vi "PIDController_Execute.vi"(4 "PID Error Tolerance":T2={"PositionTolerance"=0.001, "VelocityTolerance"=9.9e+30}, 6 "Period":dbl=0.02, 7 "PID Input Limits":T1, 8 "Reset":bool, 9 "SP-SetPoint":dbl, 10 "PV-Measurement":dbl, 11 "PID Tuning":T3={"Kp"=0.0, "Ki"=0.0, "Kd"=0.0, "MaximumIntegral"=9.9e+30, "MinimumIntegral"=-9.9e+30}) -> (0 "AtSetpoint":bool, 1 "CO-ControlOutput":dbl, 3 "out PID_CONTROLLER":T4={"Kp"=0.0, "Ki"=0.0, "Kd"=0.0, "Period"=0.0, "Max_Integral"=0.0, "Min_Integral"=0.0, "Max_Input"=0.0, "Min_Input"=0.0, "Continuous"=FALSE, "PositionError"=0.0, "VelocityError"=0.0, "PrevError"=0.0, "TotalError"=0.0, "PositionTolerance"=0.0, "VelocityTolerance"=0.0, "SetPoint"=0.0, "Kf"=0.0, "Prev_Deriv"=0.0, "Prev_Deriv 2"=0.0, "DerivativeFilter"=FALSE, "Min_Output"=-9.99e+35, "Max_Output"=9.9e+35, "Prev_F_P"=0.0, "Prev_F_P_2"=0.0, "AntiWindupActive"=FALSE} {"Prev_F_P_2" format="%16_6e"; "Prev_F_P" format="%16_6e"; "Max_Output" format="%16_6e"; "Min_Output" format="%16_6e"; "Prev_Deriv 2" format="%16_6e"; "Prev_Deriv" format="%16_6e"; "Kf" format="%16_6e"; "SetPoint" format="%16_6e"; "VelocityTolerance" format="%16_6e"; "PositionTolerance" format="%16_6e"; "TotalError" format="%16_6e"; "PrevError" format="%16_6e"; "VelocityError" format="%16_6e"; "PositionError" format="%16_6e"; "Min_Input" format="%16_6e"; "Max_Input" format="%16_6e"; "Min_Integral" format="%16_6e"; "Max_Integral" format="%16_6e"; "Period" format="%16_6e"; "Kd" format="%16_6e"; "Ki" format="%16_6e"; "Kp" format="%16_6e"})   [LabVIEW 2019, in "Trajectory_Library.lvlib"]
doc: "Convience, single call, LabVIEW function. Creates and calculates the PID controller. Call this routine periodically to calculate the newest output for the provided inputs. \n \nInputs:\n - PID Input Limits -- Cluster containing:\n - MaxInput -- (Default: 0)\n - MinInput -- (Default: 0)\n - Continous -- When True indicates that the input is continuous. (Default: False)\n - PID Tuning -- PID Tuning parameters containing:\n - Kp -- The proportional coefficient.\n - Ki -- The integral coefficient.\n - Kd -- The derivative coefficient.\n - Maximum Integral -- The maximum value of the integrator.\n - Minimum Integral -- The minimum value of the integrator.\n - PV-measurement The current measurement of the process variable. (PV)\n - SP-setpoint The new setpoint of the controller. (SP)\n - Reset -- When True, causes the PID to be reset. (Default: False)\n - Period -- Period of repeated calls in seconds. (Default: 0.020)\n - PID Error Tolerance -- Tolerances for determining \"At Setpoint\", contains:\n - Position Tolerance -- (Default: 0.001)\n - Velocity Tolerance -- (Default: 9.9E+30)\nOutputs:\n - PID_Controller -- Updated PID_Controller data cluster\n - CO-ControlOutput -- Controller output (CO) \n - AtSetpoint -- True when PV is within the specified tolerances of the SP."
uses:
  Trajectory_Library.lvlib
  PID_CONTROLLER.ctl
  PID_TUNING.ctl
  PID_INPUT_LIMITS.ctl
  PID_ERROR_TOLERANCE.ctl
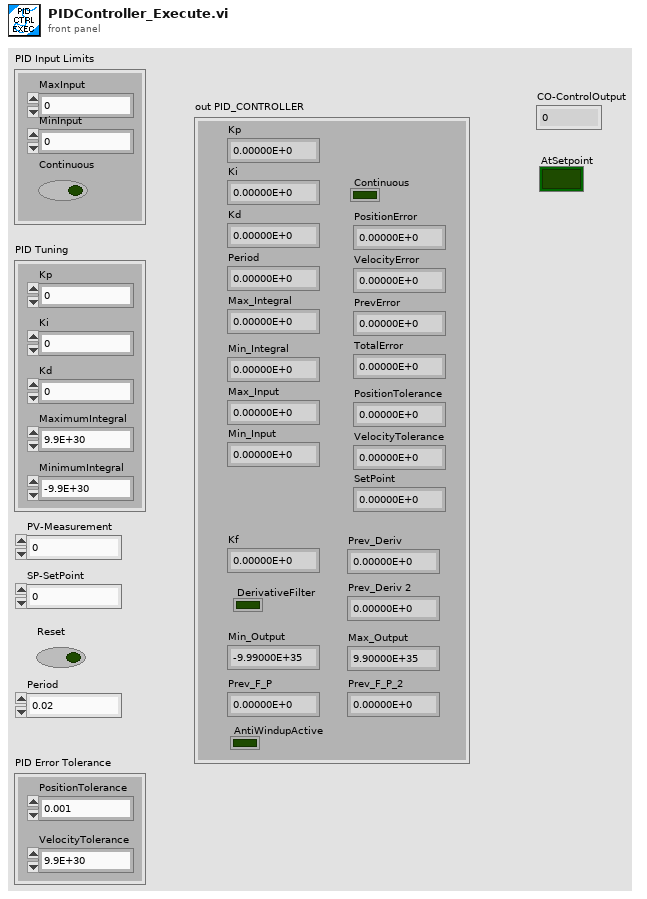
[diagram p1: front panel]
types:
  T1 = typedef "Trajectory_Library.lvlib/PID_INPUT_LIMITS.ctl" = cluster{"MaxInput":dbl, "MinInput":dbl, "Continuous":bool}
  T2 = typedef "Trajectory_Library.lvlib/PID_ERROR_TOLERANCE.ctl" = cluster{"PositionTolerance":dbl, "VelocityTolerance":dbl}
  T3 = typedef "Trajectory_Library.lvlib/PID_TUNING.ctl" = cluster{"Kp":dbl, "Ki":dbl, "Kd":dbl, "MaximumIntegral":dbl, "MinimumIntegral":dbl}
  T4 = typedef "Trajectory_Library.lvlib/PID_CONTROLLER.ctl" = cluster{"Kp":dbl, "Ki":dbl, "Kd":dbl, "Period":dbl, "Max_Integral":dbl, "Min_Integral":dbl, "Max_Input":dbl, "Min_Input":dbl, "Continuous":bool, "PositionError":dbl, "VelocityError":dbl, "PrevError":dbl, "TotalError":dbl, "PositionTolerance":dbl, "VelocityTolerance":dbl, "SetPoint":dbl, "Kf":dbl, "Prev_Deriv":dbl, "Prev_Deriv 2":dbl, "DerivativeFilter":bool, "Min_Output":dbl, "Max_Output":dbl, "Prev_F_P":dbl, "Prev_F_P_2":dbl, "AntiWindupActive":bool}
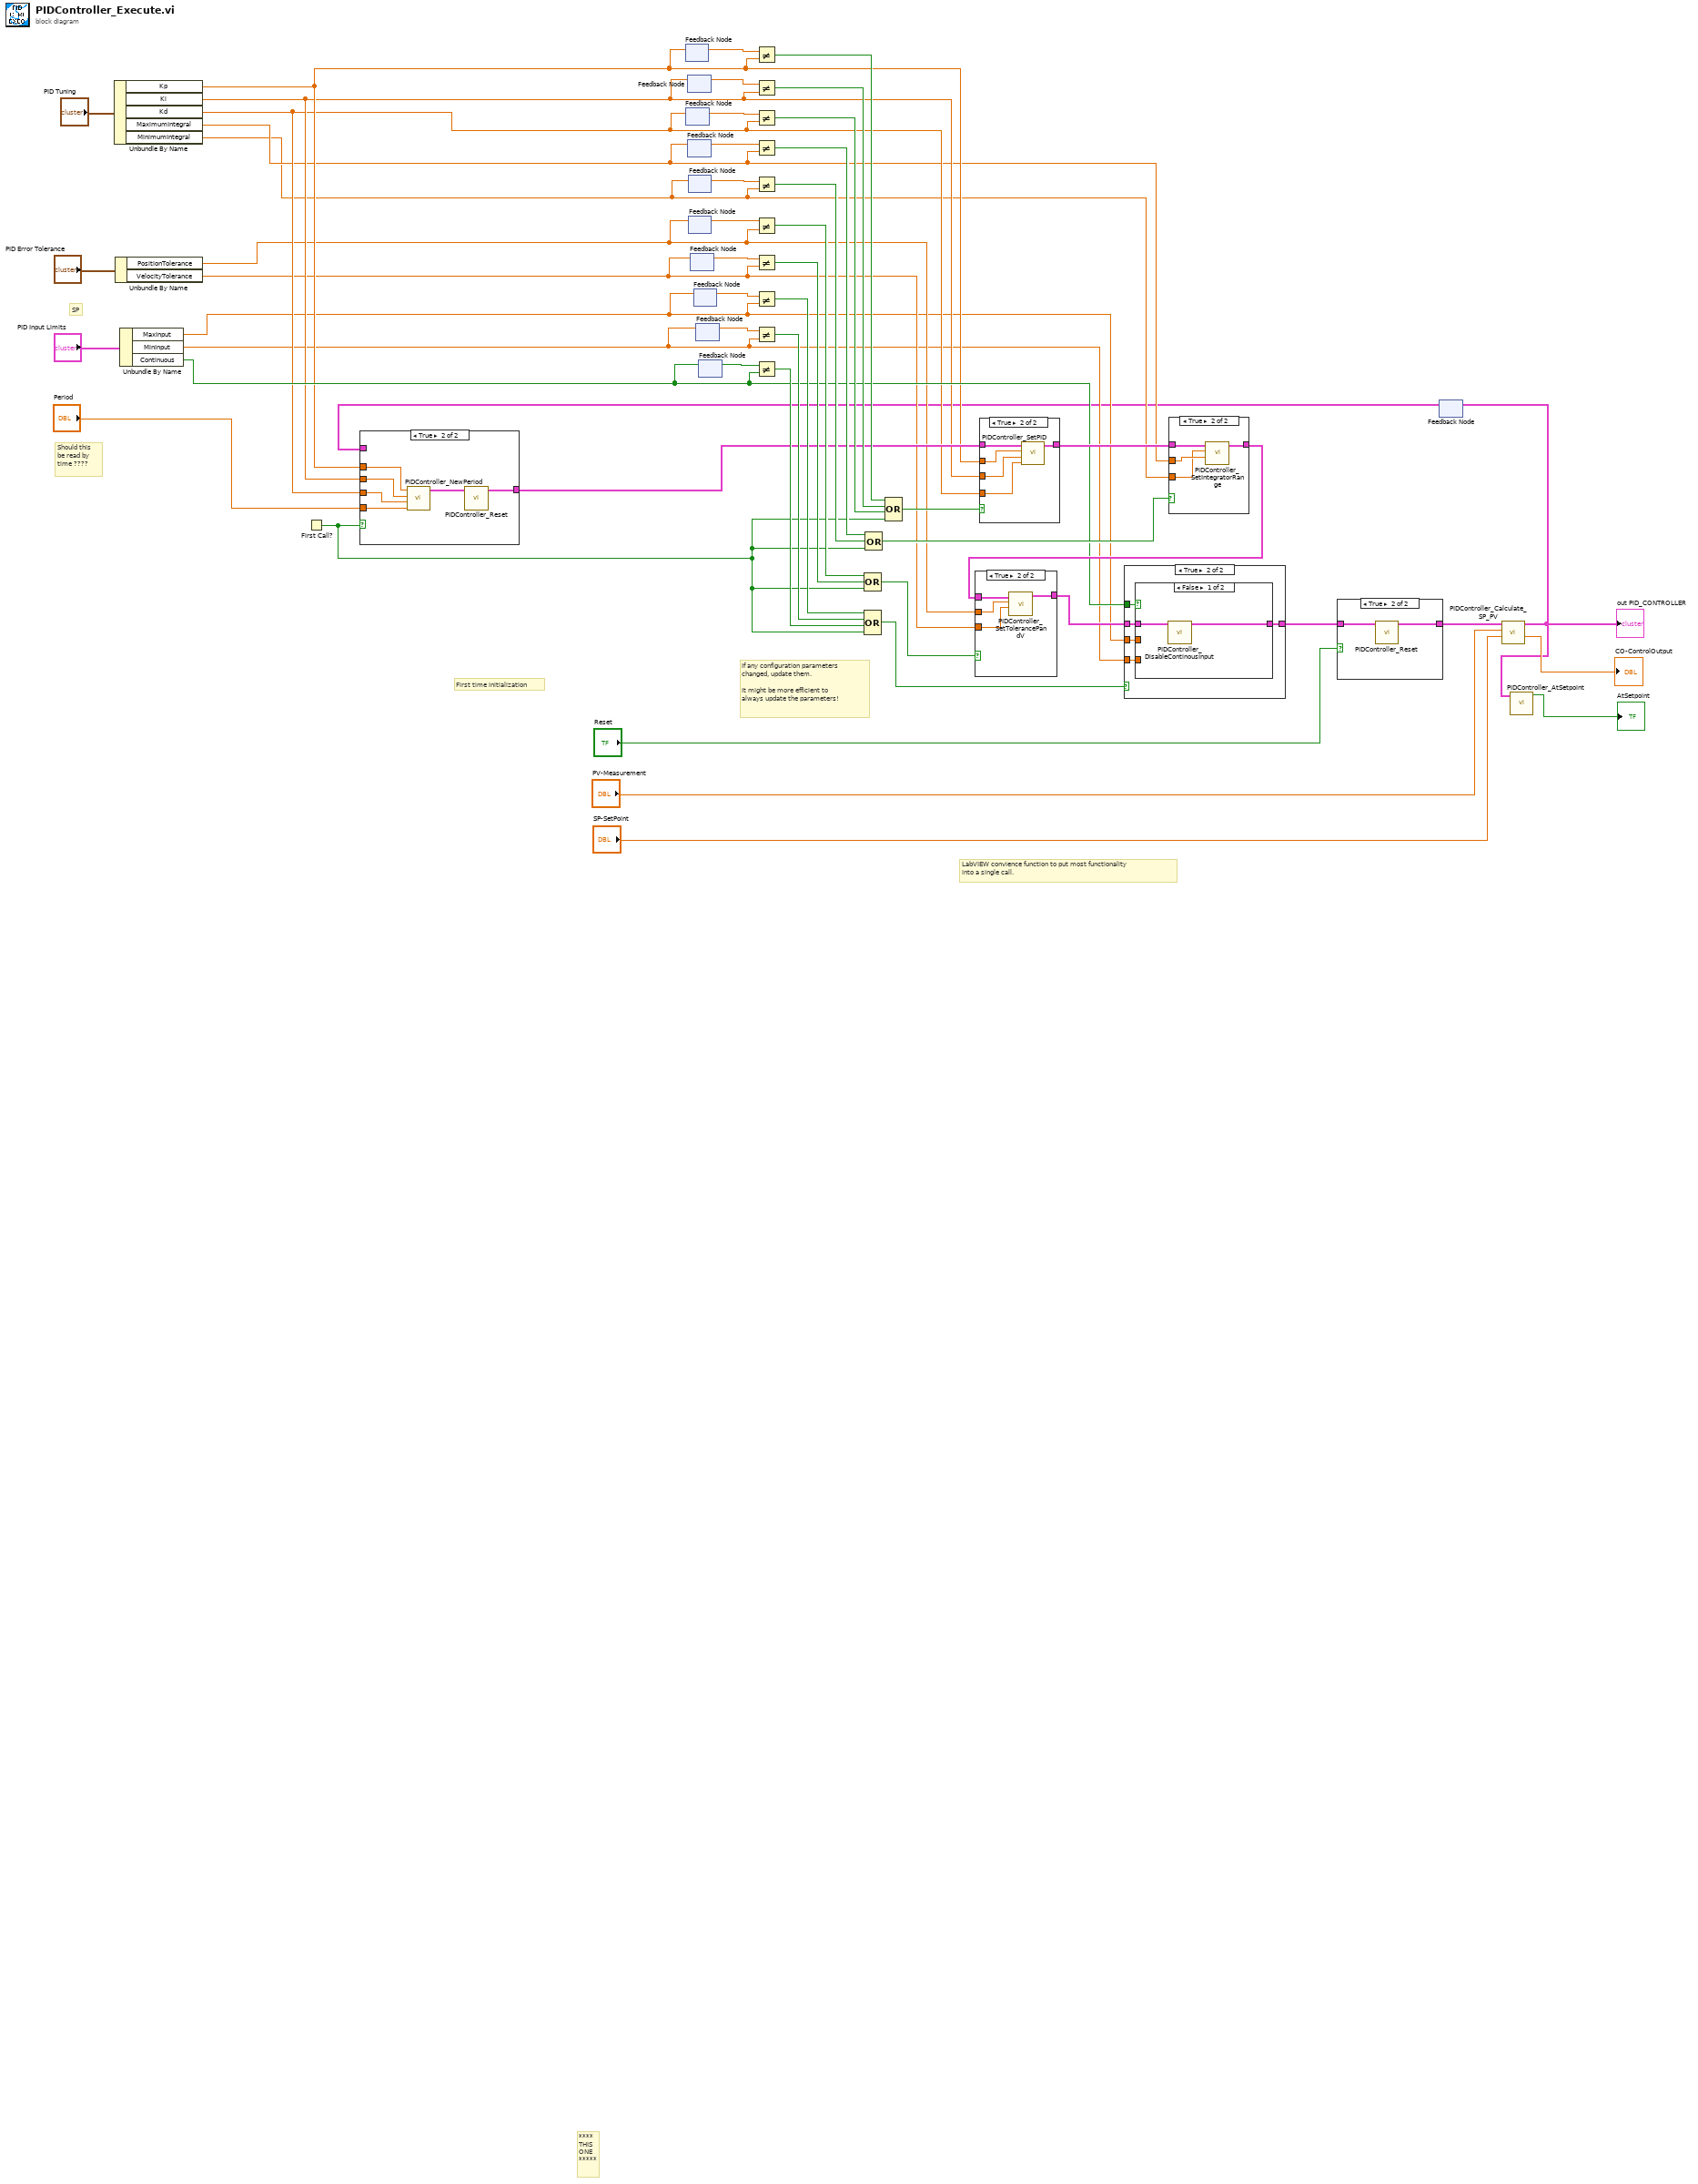
[diagram p0: block diagram]
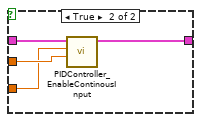
[diagram p5: hidden frame]
diagram:
  # "First time initialization"
  # "If any configuration parameters \nchanged, update them.\n\nIt might be more efficient to\nalways update the parameters!"
  # "Should this\nbe read by\ntime ????"
  # "SP"
  # "LabVIEW convience function to put most functionality\ninto a single call."
  # "****\nTHIS\nONE\n*****"
  n1 = Unbundle By Name("PID Tuning") -> ("Kp"=w21:dbl, "Ki"=w20:dbl, "Kd"=w19:dbl, "MaximumIntegral"=w18:dbl, "MinimumIntegral"=w17:dbl)
  n2 = Unbundle By Name("PID Error Tolerance") -> ("PositionTolerance"=w16:dbl, "VelocityTolerance"=w15:dbl)
  n3 = Unbundle By Name("PID Input Limits") -> ("MaxInput"=w14:dbl, "MinInput"=w13:dbl, "Continuous"=w23:bool)
  n4 = First Call?() -> (First Call?: T/F=w1:bool)
  n5 = feedback #1() -> (w12:dbl)  [unwired: 1 in]
  n6 = feedback-in #1(w21) -> ()
  n7 = feedback #2() -> (w10:dbl)  [unwired: 1 in]
  n8 = feedback-in #2(w19) -> ()
  n9 = feedback #3() -> (w11:dbl)  [unwired: 1 in]
  n10 = feedback-in #3(w20) -> ()
  n11 = feedback #4() -> (w9:dbl)  [unwired: 1 in]
  n12 = feedback-in #4(w18) -> ()
  n13 = feedback #5() -> (w8:dbl)  [unwired: 1 in]
  n14 = feedback-in #5(w17) -> ()
  n15 = feedback #6() -> (w7:dbl)  [unwired: 1 in]
  n16 = feedback-in #6(w16) -> ()
  n17 = feedback #7() -> (w6:dbl)  [unwired: 1 in]
  n18 = feedback-in #7(w15) -> ()
  n19 = feedback #8() -> (w5:dbl)  [unwired: 1 in]
  n20 = feedback-in #8(w14) -> ()
  n21 = feedback #9() -> (w4:dbl)  [unwired: 1 in]
  n22 = feedback-in #9(w13) -> ()
  n23 = feedback-in #10(w23) -> ()
  n24 = feedback #10() -> (w22:bool)  [unwired: 1 in]
  n25 = Not Equal?(x=w12, y=w21) -> (x != y?=w34:bool)
  n26 = Not Equal?(x=w11, y=w20) -> (x != y?=w35:bool)
  n27 = Not Equal?(x=w10, y=w19) -> (x != y?=w36:bool)
  n28 = Not Equal?(x=w9, y=w18) -> (x != y?=w37:bool)
  n29 = Not Equal?(x=w8, y=w17) -> (x != y?=w38:bool)
  n30 = Not Equal?(x=w7, y=w16) -> (x != y?=w39:bool)
  n31 = Not Equal?(x=w6, y=w15) -> (x != y?=w40:bool)
  n32 = Not Equal?(x=w5, y=w14) -> (x != y?=w41:bool)
  n33 = Not Equal?(x=w4, y=w13) -> (x != y?=w42:bool)
  n34 = Not Equal?(x=w22, y=w23) -> (x != y?=w43:bool)
  n35 = Compound Arithmetic op=OR(w39, w40, w1) -> (w29:bool)
  n36 = Compound Arithmetic op=OR(w41, w42, w43, w1) -> (w28:bool)
  n37 = Compound Arithmetic op=OR(w37, w38, w1) -> (w31:bool)
  n38 = Compound Arithmetic op=OR(w34, w35, w36, w1) -> (w33:bool)
  n39 = feedback #11() -> (w2:T4)  [unwired: 1 in]
  n40 = case shown="True" w1 {
    tunnel: w21 -> [_ w59]
    tunnel: w20 -> [_ w58]
    tunnel: w19 -> [_ w57]
    tunnel: "Period" -> [_ w56]
    tunnel: [w53 w55] -> w24
    tunnel: w2 -> [w53 _]
    frame False {
    }
    frame True {
      n41 = call "PIDController_NewPeriod.vi"("Period"=w56, "Kd"=w57, "Ki"=w58, "Kp"=w59) -> ("PID_CONTROLLER"=w54:T4)  [unwired: 7 in]
      n42 = call "PIDController_Reset.vi"("in PID_CONTROLLER"=w54) -> ("out PID_CONTROLLER"=w55:T4)  [unwired: 10 in]
    }
  }
  n43 = case shown="True" w33 {
    tunnel: w24 -> [w60 w65]
    tunnel: w21 -> [_ w64]
    tunnel: w20 -> [_ w63]
    tunnel: w19 -> [_ w62]
    tunnel: [w60 w61] -> w32
    frame False {
    }
    frame True {
      n44 = call "PIDController_SetPID.vi"("Kd"=w62, "Ki"=w63, "Kp"=w64, "in PID_CONTROLLER"=w65) -> ("out PID_CONTROLLER"=w61:T4)  [unwired: 7 in]
    }
  }
  n45 = case shown="True" w31 {
    tunnel: w32 -> [w66 w70]
    tunnel: w18 -> [_ w69]
    tunnel: w17 -> [_ w68]
    tunnel: [w66 w67] -> w30
    frame False {
    }
    frame True {
      n46 = call "PIDController_SetIntegratorRange.vi"("MaximumIntegral"=w69, "MinimumIntegral"=w68, "in PID_CONTROLLER"=w70) -> ("out PID_CONTROLLER"=w67:T4)  [unwired: 8 in]
    }
  }
  n47 = case shown="True" w29 {
    tunnel: w30 -> [w71 w75]
    tunnel: w16 -> [_ w74]
    tunnel: w15 -> [_ w73]
    tunnel: [w71 w72] -> w27
    frame False {
    }
    frame True {
      n48 = call "PIDController_SetTolerancePandV.vi"("VelocityTolerance"=w73, "PositionTolerance"=w74, "in PID_CONTROLLER"=w75) -> ("out PID_CONTROLLER"=w72:T4)  [unwired: 8 in]
    }
  }
  n49 = case shown="True" w28 {
    tunnel: w14 -> [_ w81]
    tunnel: w13 -> [_ w80]
    tunnel: w27 -> [w76 w79]
    tunnel: w23 -> [_ w78]
    tunnel: [w76 w77] -> w26
    frame False {
    }
    frame True {
      n50 = case shown="False" w78 {
        tunnel: w79 -> [w83 w87]
        tunnel: [w82 w86] -> w77
        tunnel: w81 -> [_ w85]
        tunnel: w80 -> [_ w84]
        frame False {
          n51 = call "PIDController_DisableContinousInput.vi"("in PID_CONTROLLER"=w83) -> ("out PID_CONTROLLER"=w82:T4)  [unwired: 10 in]
        }
        frame True {
          n52 = call "PIDController_EnableContinousInput.vi"("MaxInput"=w85, "MinInput"=w84, "in PID_CONTROLLER"=w87) -> ("out PID_CONTROLLER"=w86:T4)  [unwired: 8 in]
        }
      }
    }
  }
  n53 = case shown="True" "Reset" {
    tunnel: w26 -> [w88 w90]
    tunnel: [w88 w89] -> w25
    frame False {
    }
    frame True {
      n54 = call "PIDController_Reset.vi"("in PID_CONTROLLER"=w90) -> ("out PID_CONTROLLER"=w89:T4)  [unwired: 10 in]
    }
  }
  n55 = call "PIDController_Calculate_SP_PV.vi"("SP-SetPoint"="SP-SetPoint", "PV-Measurement"="PV-Measurement", "in PID_CONTROLLER"=w25) -> ("CO-ControlOutput"=→"CO-ControlOutput":dbl, "out PID_CONTROLLER"=w3:T4)  [unwired: 7 in]
  "out PID_CONTROLLER" <- w3
  n56 = feedback-in #11(w3) -> ()
  n57 = call "PIDController_AtSetpoint.vi"("in PID_CONTROLLER"=w3) -> ("AtSetpoint"=→"AtSetpoint":bool)  [unwired: 10 in]
